vi "Close.vi"(8 "error in (no error)":errorcluster, 11 "WebsocketStream in":refnum<class "WebsocketStream.lvclass">) -> (0 "error out":errorcluster, 3 "WebsocketStream out":refnum<class "WebsocketStream.lvclass">)   [LabVIEW 2020, in "Stream-Websocket.lvlib" / "WebsocketStream.lvclass"]
uses:
  WebsocketStream.lvclass
  Client Command.ctl
  Stream-Websocket.lvlib
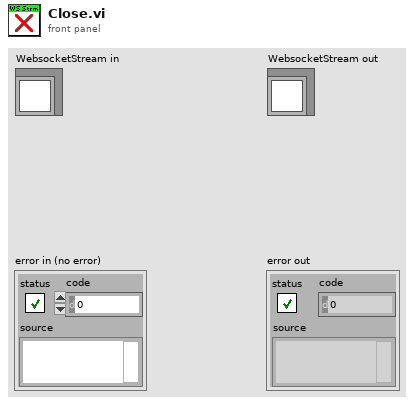
[diagram p1: front panel]
types:
  T1 = typedef "Stream-Websocket.lvlib/Client Command.ctl" = enum16{"Connect", "Close", "Shutdown", "Reconnect"}
  T2 = typedef "Stream-Websocket.lvlib/WebsocketStream.lvclass/Ref Data.ctl" = cluster{"Command Queue":refnum<queue>, "Closing":bool}
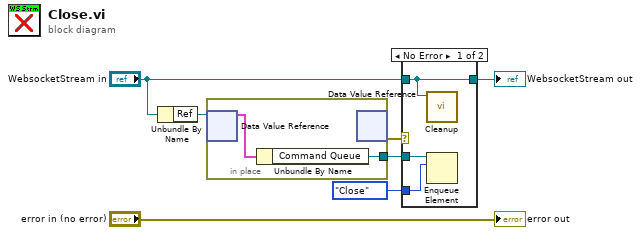
[diagram p0: block diagram]
diagram:
  n1 = Unbundle By Name("WebsocketStream in") -> ("Ref"=w6:refnum<data-value>)
  n2 = in-place {
    in-place-border: [w8] -> w5
    n3 = in-place-dvr #1(w6) -> (w9:T2)  [unwired: 1 out]
    n4 = Unbundle By Name(w9) -> ("Command Queue"=w8:refnum<queue>)
    n5 = in-place-dvr #1() -> (w4:errorcluster)  [unwired: 1 in, 1 out]
  }
  n6 = case shown="No Error" w4 {
    tunnel: w5 -> [w12 _]
    tunnel: "WebsocketStream in" -> [w10 w13]
    tunnel: Client_Command."Close" ("element") -> [w11 _]
    tunnel: [w10 w13] -> w1
    frame No Error {
      n7 = call "Cleanup.vi"("WebsocketStream in"=w10) -> ()  [unwired: 10 in, 1 out]
      n8 = Enqueue Element(queue=w12, element=w11) -> ()  [unwired: 2 in, 3 out]
    }
    frame Error {
    }
  }
  "WebsocketStream out" <- w1
  "error out" <- "error in (no error)"
